vi "Untitled 5 (SubVI).vi"(10 "Numeric":i32=8, 11 "String":string) -> (3 "Boolean array":bool[][](array[boolean]))   [LabVIEW 2016]
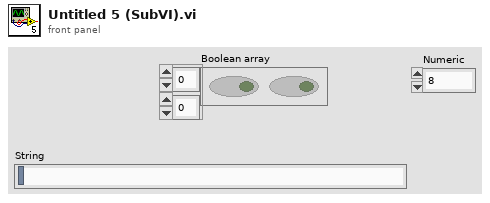
[diagram p1: front panel]
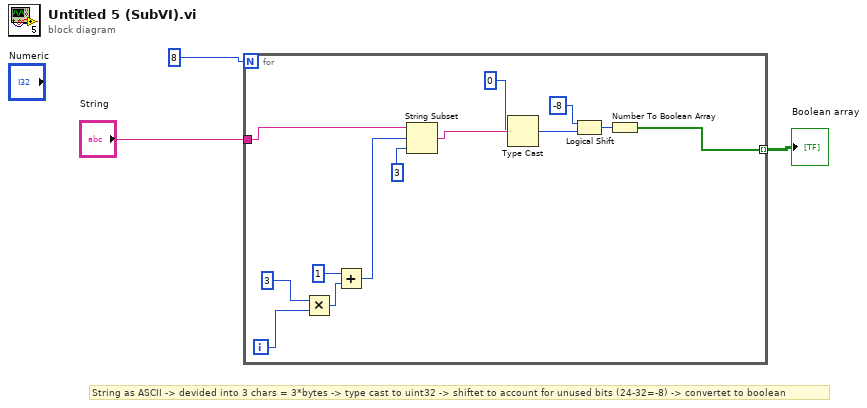
[diagram p0: block diagram]
diagram:
  # "String as ASCII -> devided into 3 chars = 3*bytes -> type cast to uint32 -> shiftet to account for unused bits (24-32=-8) -> convertet to boolean"
  n1 = for {
    N: 8 -> [_]
    tunnel: "String" -> [w16]
    tunnel: [w12] -> w3 mode=indexing
    i -> [w14]
    n2 = Multiply(x=3, y=w14) -> (x*y=w11:i32)
    n3 = Add(x=1, y=w11) -> (x+y=w9:i32)
    n4 = String Subset(string=w16, offset (0)=w9, length (rest)=3 ("length (rest)")) -> (substring=w8:string)
    n5 = Type Cast(type=u32 0, x=w8) -> (*(type *) &x=w6:u32)
    n6 = Logical Shift(y=i16 -8, x=w6) -> (x << y=w4:u32)
    n7 = Number To Boolean Array(number=w4) -> (Boolean array=w12:bool[])
  }
  "Boolean array" <- w3
